vi "Protocol.Cleanup.vi"(8 "error in (no error)":errorcluster, 11 "J1939 Main Configuration":T1 {"Stream Refs"."Port Settings"."FD ISO Mode" items=["ISO", "Non ISO", "ISO Legacy"]; "Stream Refs"."Port Settings"."Termination" items=["Off", "On"]; "Stream Refs"."Port Settings"."Mode" items=["CAN 2.0", "CAN FD", "CAN FD+BRS"]}) -> (0 "error out":errorcluster)   [LabVIEW 2019, in "J1939 Addon Engine.lvlib"]
uses:
  J1939 Addon Engine.lvlib
  Types/Protocol.Configuration.ctl
  <vilib>/NI/NI VeriStand Addon Network Comm/Engine/VeriStand Comm.lvclass
  <vilib>/NI/NIVS Inline Async API/_VS Inline Async API/Process/Process.lvclass
  Types/Protocol.Refs.ctl
  Support Libraries/J1939 Utilities/Types/CAN Outgoing Message Cluster.ctl
  Types/Protocol.RQST Lookup Table Reference.ctl
  Types/Protocol.Address Table Reference.ctl
  Types/Protocol.XNET Settings.ctl
  <vilib>/NI/NIVS Inline Async API/_Data Access Engine/Data Access Engine/Types/Read.DVR.ctl
  <vilib>/NI/NIVS Inline Async API/_Data Access Engine/Access Type Classes/Read/Read.lvclass
  <vilib>/NI/NIVS Inline Async API/_Data Access Engine/Data Access Engine/Types/Write.DVR.ctl
  <vilib>/NI/NIVS Inline Async API/_Data Access Engine/Access Type Classes/Write/Write.lvclass
  Types/CounterAndProtectionFrames.ctl
  SubModules/Frame-Protection-Support/Source/Engine/Types/RT Frame Settings.ctl
  SubModules/Frame-Protection-Support/Source/Shared/Types/Exported Frame Type.ctl
  SubModules/Frame-Protection-Support/Source/Engine/Types/RT Protection Configuration.ctl
  SubModules/Frame-Protection-Support/Source/Shared/Types/Protection Type.ctl
  SubModules/Frame-Protection-Support/Source/Shared/Types/XNET Signal Configuration.ctl
  SubModules/Frame-Protection-Support/Source/Shared/Types/Exported Counter Settings.ctl
  SubModules/Frame-Protection-Support/Source/Shared/Types/Exported Event Trigger Type.ctl
  SubModules/CAN-Streaming-Support/Source/Addon/Addon Engine/Types/Engine Stream Refs.ctl
  SubModules/CAN-Streaming-Support/Source/Addon/Addon Shared/Types/Direction Filter.ctl
  SubModules/CAN-Streaming-Support/Source/Addon/Addon Shared/Types/Type Filter.ctl
  SubModules/CAN-Streaming-Support/Source/Addon/Addon Shared/Types/Filter Parameters.ctl
  SubModules/CAN-Streaming-Support/Source/Addon/Addon Engine/Types/Engine Stream Port Settings.ctl
  <vilib>/Utility/SystemLogging/Write to System Log.vi
  Support Libraries/J1939 Utilities/J1939 Utilities.lvlib
  <vilib>/NI/NIVS Inline Async API/_Data Access Engine/Data Access Engine/Data Access Engine.lvclass
  SubModules/Frame-Protection-Support/Source/Engine/Protection and Counter Support Engine.lvlib
  SubModules/Frame-Protection-Support/Source/Shared/Protection and Counter Support Shared.lvlib
  SubModules/CAN-Streaming-Support/Source/Addon/Addon Shared/CAN Stream Support Shared.lvlib
  SubModules/CAN-Streaming-Support/Source/Addon/Addon Engine/CAN Stream Support Engine.lvlib
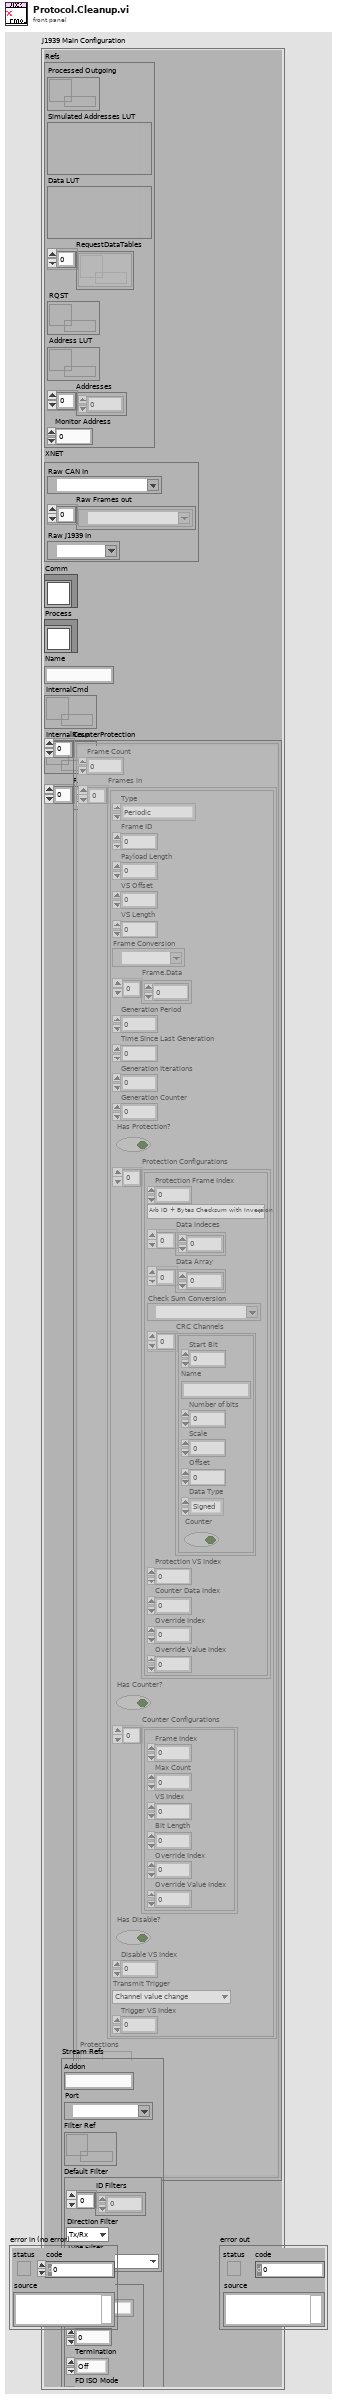
[diagram p1: front panel]
types:
  T1 = typedef "J1939 Addon Engine.lvlib/Protocol.Configuration.ctl" = cluster{"Refs":T2, "XNET":T5, "Comm":refnum<class "VeriStand Comm.lvclass">, "Process":refnum<class "Process.lvclass">, "Name":string, "InternalCmd":T6, "InternalResp":T7, "Resp.Data":dbl[], "CounterProtection":T8[], "Stream Refs":T16}
  T2 = typedef "J1939 Addon Engine.lvlib/Protocol.Refs.ctl" = cluster{"Processed Outgoing":refnum<queue>, "Simulated Addresses LUT":variant, "Data LUT":variant, "RequestDataTables":refnum<k33>[], "RQST":T3, "Address LUT":T4, "Addresses":u8[], "Monitor Address":u8}
  T3 = typedef "J1939 Addon Engine.lvlib/Protocol.RQST Lookup Table Reference.ctl" = refnum<data-value>
  T4 = typedef "J1939 Addon Engine.lvlib/Protocol.Address Table Reference.ctl" = refnum<data-value>
  T5 = typedef "J1939 Addon Engine.lvlib/Protocol.XNET Settings.ctl" = cluster{"Raw CAN In":refnum<k21>, "Raw Frames out":refnum<k21>[], "Raw J1939 In":refnum<k21>}
  T6 = typedef "Data Access Engine.lvlib/Data Access Engine.lvclass/Read.DVR.ctl" = refnum<data-value>
  T7 = typedef "Data Access Engine.lvlib/Data Access Engine.lvclass/Write.DVR.ctl" = refnum<data-value>
  T8 = typedef "J1939 Addon Engine.lvlib/CounterAndProtectionFrames.ctl" = cluster{"Frame Count":i32, "Frames in":T9[], "Protections":T7, "Signals":T6, "Overrides":T6}
  T9 = typedef "Protection and Counter Support Engine.lvlib/RT Frame Settings.ctl" = cluster{"Type":T10, "Frame ID":u32, "Payload Length":u32, "VS Offset":i32, "VS Length":i32, "Frame Conversion":refnum<k21>, "Frame.Data":dbl[], "Generation Period":u32, "Time Since Last Generation":u32, "Generation Iterations":u32, "Generation Counter":u32, "Has Protection?":bool, "Protection Configurations":T11[], "Has Counter?":bool, "Counter Configurations":T14[], "Has Disable?":bool, "Disable VS Index":i32, "Transmit Trigger":T15, "Trigger VS Index":i32}
  T10 = typedef "Protection and Counter Support Shared.lvlib/Exported Frame Type.ctl" = enum16{"Periodic", "Event", "Periodic/Event"}
  T11 = typedef "Protection and Counter Support Engine.lvlib/RT Protection Configuration.ctl" = cluster{"Protection Frame Index":i32, "Protection Type":T12, "Data Indeces":i32[], "Data Array":dbl[], "Check Sum Conversion":refnum<k21>, "CRC Channels":T13[], "Protection VS Index":i32, "Counter Data Index":i32, "Override Index":i32, "Override Value Index":i32}
  T12 = typedef "Protection and Counter Support Shared.lvlib/Protection Type.ctl" = enum16{"Arb ID + Bytes Checksum with Inversion", "Arb ID + Bytes CRC with Inversion", "Reversed Raw Signal Checksum with Inversion", "Concatenated Two's Compliment"}
  T13 = typedef "Protection and Counter Support Shared.lvlib/XNET Signal Configuration.ctl" = cluster{"Start Bit":i32, "Name":string, "Number of bits":i32, "Scale":dbl, "Offset":dbl, "Data Type":u32, "Counter":bool}
  T14 = typedef "Protection and Counter Support Shared.lvlib/Exported Counter Settings.ctl" = cluster{"Frame Index":i32, "Max Count":dbl, "VS Index":i32, "Bit Length":i64, "Override Index":i32, "Override Value Index":i32}
  T15 = typedef "Protection and Counter Support Shared.lvlib/Exported Event Trigger Type.ctl" = enum16{"Channel value change", "Trigger channel (not zero)", "Channel value change or trigger channel (not zero)", "Trigger channel (any value change)", "Channel value change or trigger channel (any value change)"}
  T16 = typedef "CAN Stream Support Engine.lvlib/Engine Stream Refs.ctl" = cluster{"Addon":string, "Port":refnum<k21>, "Filter Ref":refnum<data-value>, "Default Filter":T17, "Port Settings":T20}
  T17 = typedef "CAN Stream Support Shared.lvlib/Filter Parameters.ctl" = cluster{"ID Filters":u32[], "Direction Filter":T18, "Type Filter":T19}
  T18 = typedef "CAN Stream Support Shared.lvlib/Direction Filter.ctl" = enum16{"Tx/Rx", "Rx", "Tx"}
  T19 = typedef "CAN Stream Support Shared.lvlib/Type Filter.ctl" = enum16{"All", "CAN Data", "CAN Remote", "CAN Bus Error", "CAN 2.0 Data", "CAN FD Data", "CAN FD+BRS Data", "J1939 Data", "Delay", "Log Trigger", "Start Trigger"}
  T20 = typedef "CAN Stream Support Engine.lvlib/Engine Stream Port Settings.ctl" = cluster{"Mode":u32, "Baud Rate":u64, "Termination":u32, "FD ISO Mode":u32, "FD Baud Rate":u64}
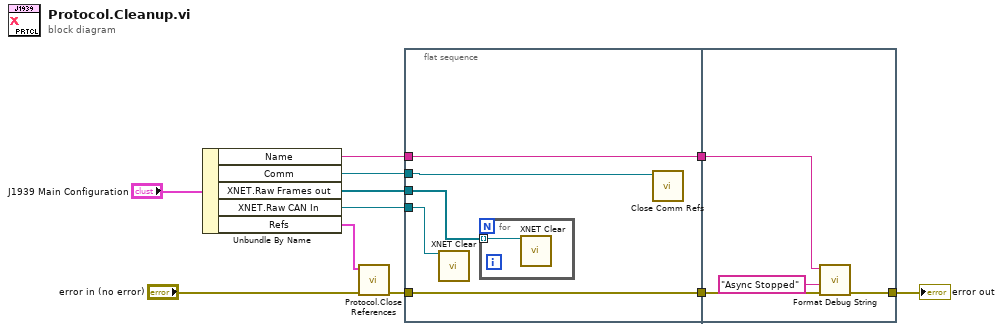
[diagram p0: block diagram]
diagram:
  n1 = Unbundle By Name("J1939 Main Configuration") -> ("Name"=w1:string, "Comm"=w2:refnum<class "VeriStand Comm.lvclass">, "XNET.Raw Frames out"=w3:refnum<k21>[], "XNET.Raw CAN In"=w4:refnum<k21>, "Refs"=w5:T2)
  n2 = call "Protocol.Close References.vi"("error in"="error in (no error)", "J1939 Cluster"=w5) -> ("error out"=w8:errorcluster)  [unwired: 9 in]
  n3 = flat-sequence {
    tunnel: w8 -> [w16]
    tunnel: [w16] -> w11
    tunnel: [w13] -> w10
    tunnel: w4 -> [w15]
    tunnel: w3 -> [w14]
    tunnel: w2 -> [w12]
    tunnel: w1 -> [w13]
    tunnel: [w20] -> w9
    tunnel: w11 -> [w19]
    tunnel: w10 -> [w18]
    frame #0 {
      n4 = call <vilib>:"XNET Clear.vi"("session in"=w15) -> ()  [unwired: 14 in, 1 out]
      n5 = for {
        tunnel: w14 -> [w17] mode=indexing
        n6 = call <vilib>:"XNET Clear.vi"("session in"=w17) -> ()  [unwired: 14 in, 1 out]
      }
      n7 = call <vilib>:"Close Comm Refs.vi"("Comm.lvclass"=w12) -> ()  [unwired: 10 in, 1 out]
    }
    frame #1 {
      n8 = call "Format Debug String.vi"("error in (no error)"=w19, "State"="Async Stopped", "Name"=w18) -> ("error out"=w20:errorcluster)  [unwired: 8 in]
    }
  }
  "error out" <- w9
